vi "FGV_Timer.vi"(6 "TimerAction (TimerElapsed)":T1=enum."TimerElapsed", 8 "error in (no error)":errorcluster, 11 "TimeToElapse (10) (s)":dbl=10.0) -> (0 "error out":errorcluster, 2 "Time Elapsed?":bool, 3 "Time Elapsed (s)":dbl)   [LabVIEW 2020]
doc: "This Vi checks if the Time to Elapse has actually Elapsed and returns Time Elapsed."
uses:
  #typedef_TimerAction.ctl
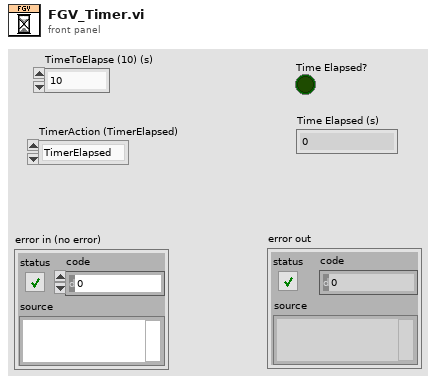
[diagram p1: front panel]
types:
  T1 = typedef "#typedef_TimerAction.ctl" = enum16{"Reset", "TimerElapsed"}
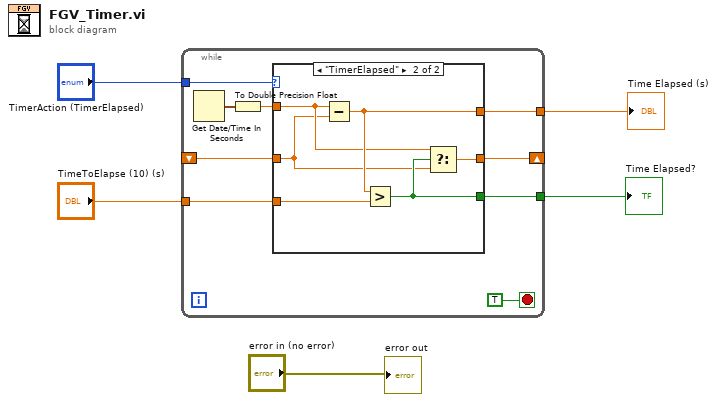
[diagram p0: block diagram]
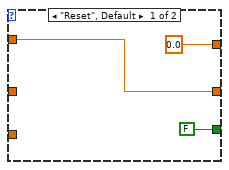
[diagram p2: hidden frame]
diagram:
  n1 = while {
    shift-right: [w11] -> _
    shift-left: _ -> [w10]
    tunnel: "TimerAction (TimerElapsed)" -> [w14]
    tunnel: [w9] -> w4
    tunnel: [w7] -> w2
    tunnel: "TimeToElapse (10) (s)" -> [w6]
    stop <- TRUE stop-if-true
    n2 = Get Date/Time In Seconds() -> (seconds since 1Jan1904=w13:timestamp)
    n3 = To Double Precision Float(number=w13) -> (double precision float=w12:dbl)
    n4 = case shown="\"TimerElapsed\"" w14 {
      tunnel: w12 -> [w17 w19]
      tunnel: [w17 w21] -> w11
      tunnel: w10 -> [_ w18]
      tunnel: [0.0 w22] -> w9
      tunnel: w6 -> [_ w23]
      tunnel: [FALSE w20] -> w7
      frame "Reset", Default {
      }
      frame "TimerElapsed" {
        n5 = Subtract(x=w19, y=w18) -> (x-y=w22:dbl)
        n6 = Greater?(x=w22, y=w23) -> (0:w20:bool)
        n7 = Select(t=w19, s=w20, f=w18) -> (s? t:f=w21:dbl)
      }
    }
  }
  "Time Elapsed (s)" <- w4
  "Time Elapsed?" <- w2
  "error out" <- "error in (no error)"
